vi "FT_Read_String_Data.vi"(0 "Handle":u32, 1 "Bytes To Read":u32) -> (2 "FT_Status":u32, 3 "Read Data":string, 4 "Bytes Read":u32)   [LabVIEW 2016]
uses:
  FTD2XX.dll
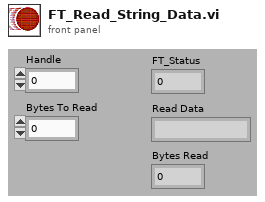
[diagram p1: front panel]
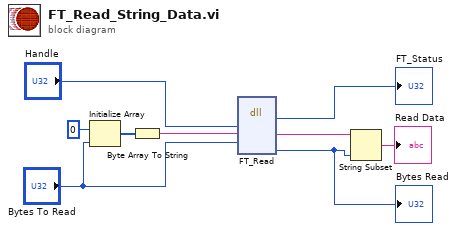
[diagram p0: block diagram]
diagram:
  n1 = Initialize Array(u8 0, "Bytes To Read") -> (w6:u8[])
  n2 = Byte Array To String(unsigned byte array=w6) -> (string=w5:string)
  n3 = dll-call lib="FTD2XX.dll" fn="FT_Read"("Handle"="Handle", "Buffer"=w5, "BytesToRead"="Bytes To Read") -> ("FT_Status"=→"FT_Status":u32, "Buffer"=w2:string, "BytesReturned"=w1:u32)  [unwired: 6 in, 2 out]
  "Bytes Read" <- w1
  n4 = String Subset(string=w2, length (rest)=w1) -> (substring=→"Read Data":string)  [unwired: 1 in]
